vi "Init Options.vi"(8 "error in (no error)":errorcluster, 11 "VISA Resource Name":refnum<visa-resource-name>) -> (0 "error out":errorcluster, 3 "VISA Resource Name Out":refnum<visa-resource-name>)   [LabVIEW 2010, in "Tektronix TDS 3000 Series.lvlib"]
doc: "This VI resets all values that the TKTDS3K reset VI does not cover."
uses:
  <instrlib>/Tektronix TDS 3000 Series/Tektronix TDS 3000 Series.lvlib
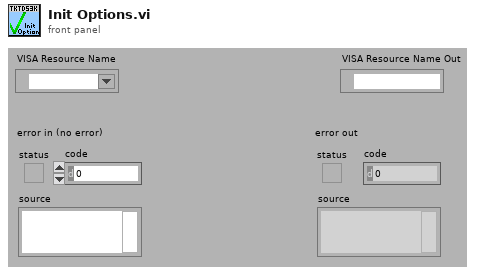
[diagram p1: front panel]
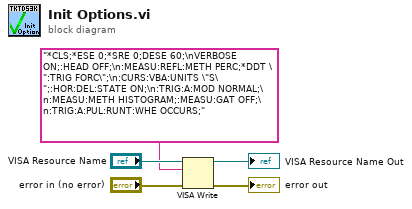
[diagram p0: block diagram]
diagram:
  n1 = VISA Write(VISA resource name="VISA Resource Name", write buffer="*CLS;*ESE 0;*SRE 0;DESE 60;\nVERBOSE ON;:HEAD OFF;\n:MEASU:REFL:METH PERC;*DDT \":TRIG FORC\";\n:CURS:VBA:UNITS \"S\";:HOR:DEL:STATE ON;\n:TRIG:A:MOD NORMAL;\n:MEASU:METH HISTOGRAM;:MEASU:GAT OFF;\n:TRIG:A:PUL:RUNT:WHE OCCURS;", error in (no error)="error in (no error)") -> (VISA resource name out=→"VISA Resource Name Out":refnum<visa-resource-name>, error out=→"error out":errorcluster)  [unwired: 1 out]
